vi "Call Commands.vi"(10 "Iterations":i32, 11 "Commands":cluster{"Time (s)":dbl, T1, bool}[](array[cluster])) -> ()   [LabVIEW 2020]
uses:
  <vilib>/picture/picture.llb/imagedata.ctl
  submodules/bordeaux-pathinator/Bordeaux/Types/Single Cmd Info.ctl
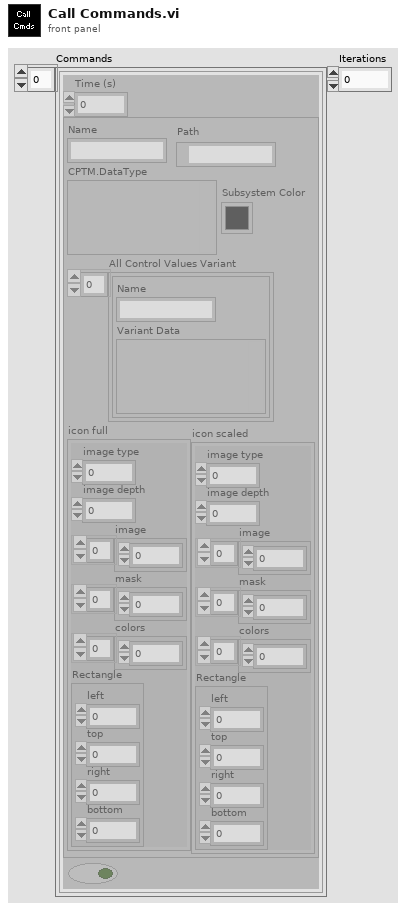
[diagram p1: front panel]
types:
  T1 = typedef "Single Cmd Info.ctl" = cluster{"Name":string, "CPTM.DataType":variant, "All Control Values Variant":cluster{"Name":string, "Variant Data":variant}[], "icon full":T2, "icon scaled":T2, "Path":path, "Subsystem Color":u32}
  T2 = typedef "imagedata.ctl" = cluster{"image type":i32, "image depth":i32, "image":u8[], "mask":u8[], "colors":u32[], "Rectangle":cluster{"left":i16, "top":i16, "right":i16, "bottom":i16}}
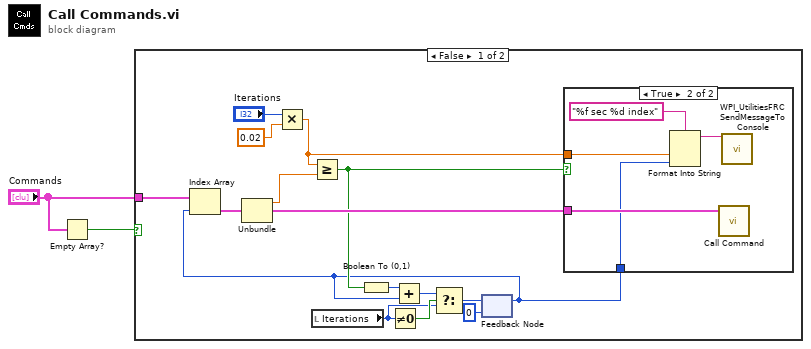
[diagram p0: block diagram]
diagram:
  n1 = Empty Array?(array="Commands") -> (empty?=w2:bool)
  n2 = case shown="False" w2 {
    tunnel: "Commands" -> [w17 _]
    frame False {
      n3 = Multiply(x="Iterations", y=0.02) -> (x*y=w11:dbl)
      n4 = local read "Iterations"() -> (w6:i32)
      n5 = Not Equal To 0?(x=w6) -> (x != 0?=w7:bool)
      n6 = feedback #1(0 ("Iterations")) -> (w3:i32)
      n7 = Index Array(array=w17, index=w3) -> (element=w16:cluster{"Time (s)":dbl, T1, bool})
      n8 = Unbundle(w16) -> ("Time (s)"=w12:dbl, w15:T1)  [unwired: 1 out]
      n9 = Greater Or Equal?(x=w11, y=w12) -> (x >= y?=w10:bool)
      n10 = Boolean To (0,1)(Boolean=w10) -> (0, 1=w9:i16)
      n11 = Add(x=w9, y=w3) -> (x+y=w8:i32)
      n12 = Select(t=w8, s=w7, f=w6) -> (s? t:f=w5:i32)
      n13 = feedback-in #1(w5) -> ()
      n14 = case shown="True" w10 {
        tunnel: w15 -> [_ w22]
        tunnel: w11 -> [_ w19]
        tunnel: w3 -> [_ w18]
        frame False {
        }
        frame True {
          n15 = Format Into String(format string="%f sec %d index", w19, w18) -> (resulting string=w20:string)  [unwired: 2 in, 1 out]
          n16 = call "Call Command.vi"("Command"=w22) -> ()  [unwired: 11 in]
          n17 = call <vilib>:"WPI_UtilitiesFRC SendMessageToConsole.vi"("Message"=w20) -> ()  [unwired: 14 in, 1 out]
        }
      }
    }
    frame True {
    }
  }
